vi "main.vi"   [LabVIEW 2020]
uses:
  api message.ctl
  api states.ctl
  user events.ctl
types:
  T1 = typedef "user events.ctl" = cluster{"stop":refnum<user-event>, "API message":refnum<user-event>}
  T2 = typedef "api message.ctl" = cluster{"API States":T3, "payload":variant}
  T3 = typedef "api states.ctl" = enum16{"stop", "say"}
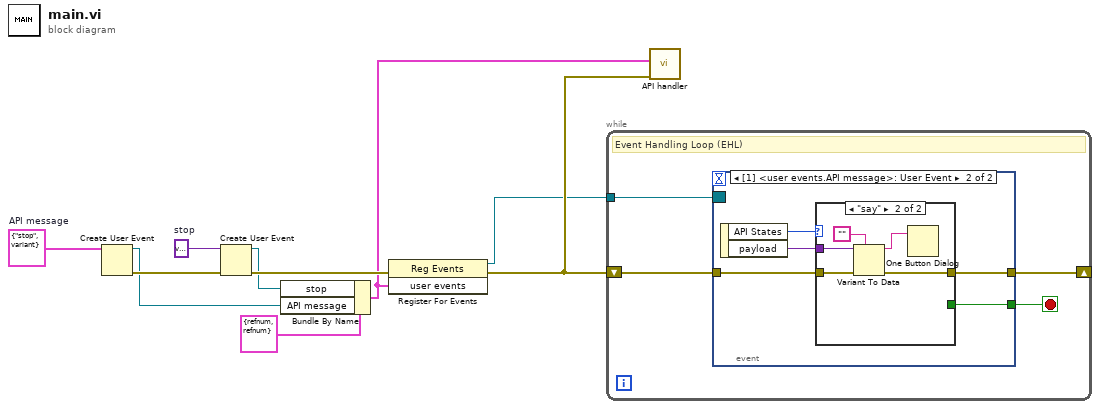
[diagram p0: block diagram]
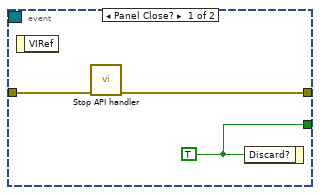
[diagram p2: hidden frame]
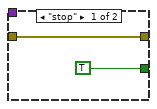
[diagram p3: hidden frame]
diagram:
  w8 = T2 {"API States"=enum."stop", "payload"=variant}  # API message
  w9 = variant  # stop
  n1 = Create User Event(user event datatype=w8) -> (user event=w5:refnum<user-event>, error out=w7:errorcluster)  [unwired: 1 in]
  n2 = Create User Event(user event datatype=w9, error in=w7) -> (user event=w6:refnum<user-event>, error out=w10:errorcluster)
  n3 = Bundle By Name(cluster=T1 {"stop"=refnum, "API message"=refnum} ("user events"), "stop"=w6, "API message"=w5) -> (w3:T1)
  n4 = register-events(error in=w10, w3) -> (reference out=w1:refnum<event-registration>, error out=w2:errorcluster)  [unwired: 1 in]
  n5 = while {
    tunnel: w1 -> [w13]
    shift-right: [w11] -> _
    shift-left: w2 -> [w12]
    stop <- w14 stop-if-true
    # "Event Handling Loop (EHL)"
    n6 = event shown="[1] <user events.API message>: User Event" {
      selector: w13 -> [_ _]
      dyn-events: _ -> [_ _]
      timeout: _ -> [_ _]
      tunnel: [w17 w19] -> w14
      tunnel: w12 -> [w16 w21]
      tunnel: [w15 w20] -> w11
      event Panel Close? {
        w17 = TRUE
        n7 = event-data() -> ()  [unwired: 1 in, 1 out]
        n8 = call "Stop API handler.vi"("error in (no error)"=w16) -> ("error out"=w15:errorcluster)  [unwired: 10 in]
        n9 = event-data("Discard?"=w17) -> ()  [unwired: 1 in, 1 out]
      }
      event User Event {
        n10 = event-data() -> ("API States"=w22:T3, "payload"=w18:variant)  [unwired: 1 in]
        n11 = case shown="\"say\"" w22 {
          tunnel: w21 -> [w24 w29]
          tunnel: [w24 w28] -> w20
          tunnel: [TRUE _] -> w19
          tunnel: w18 -> [_ w27]
          frame "stop" {
          }
          frame "say" {
            n12 = Variant To Data(error in=w29, type="", Variant=w27) -> (data=w25:string, error out=w28:errorcluster)
            n13 = One Button Dialog(message=w25) -> ()  [unwired: 1 in, 1 out]
          }
        }
      }
    }
  }
  n14 = call "API handler.vi"("error in (no error)"=w2, "user events"=w3) -> ()  [unwired: 9 in, 1 out]
